vi "Similarities_to_colour_grid.vi"(11 "Array in":dbl[][](array[numeric])) -> (3 "Array out":u32[][](array[numeric]))   [LabVIEW 2016]
uses:
  <vilib>/Analysis/baseanly.llb/Mean (DBL).vi
  <vilib>/Analysis/NI_AALBase.lvlib
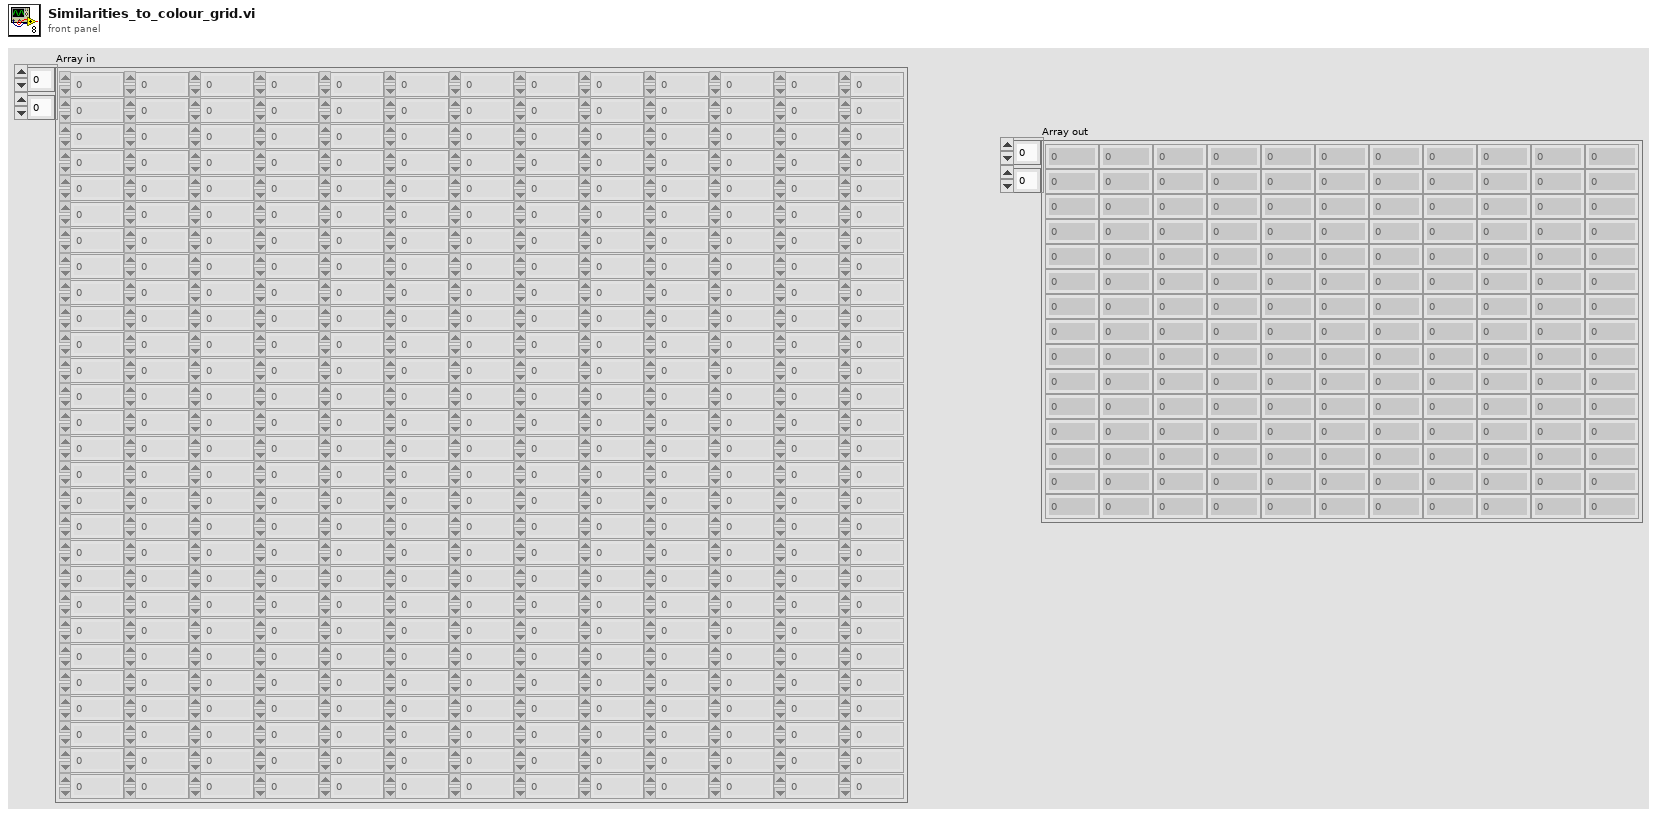
[diagram p1: front panel]
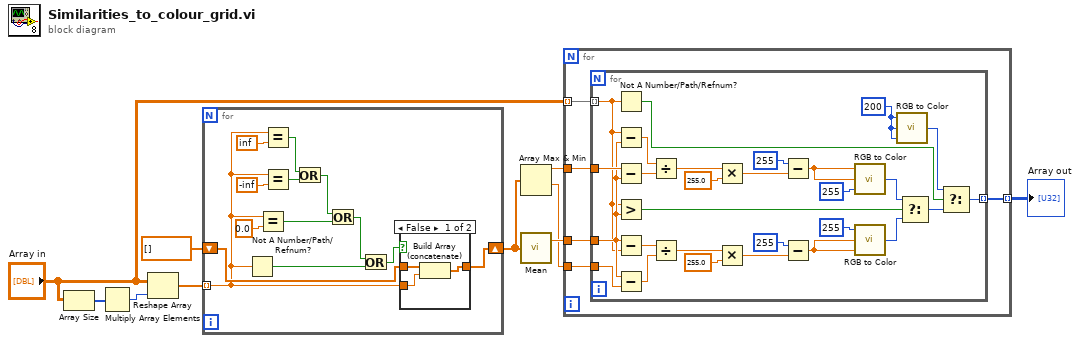
[diagram p0: block diagram]
diagram:
  n1 = Array Size(array="Array in") -> (size(s)=w2:i32[])
  n2 = Multiply Array Elements(1:w2) -> (0:w1:i32)
  n3 = Reshape Array("Array in", w1) -> (w6:dbl[])
  n4 = for {
    tunnel: w6 -> [w14] mode=indexing
    shift-right: [w21] -> w4
    shift-left: dbl[] [] ("output array") -> [w22]
    n5 = Not A Number/Path/Refnum?(number/path/refnum=w14) -> (NaN/Path/Refnum?=w13:bool)
    n6 = Equal?(x=w14, y=0.0) -> (x = y?=w16:bool)
    n7 = Equal?(x=w14, y=inf) -> (x = y?=w19:bool)
    n8 = Equal?(x=w14, y=-inf) -> (x = y?=w18:bool)
    n9 = Or(x=w19, y=w18) -> (x .or. y?=w17:bool)
    n10 = Or(x=w17, y=w16) -> (x .or. y?=w12:bool)
    n11 = Or(x=w12, y=w13) -> (x .or. y?=w11:bool)
    n12 = case shown="False" w11 {
      tunnel: w14 -> [w25 _]
      tunnel: w22 -> [w26 w27]
      tunnel: [w24 w27] -> w21
      frame False {
        n13 = Build Array (concatenate)(w26, w25) -> (w24:dbl[])
      }
      frame True {
      }
    }
  }
  n14 = Array Max & Min(array=w4) -> (max value=w9:dbl, min value=w8:dbl)  [unwired: 2 out]
  n15 = call-poly <vilib>:"Mean.vi"("X"=w4) -> ("mean"=w10:dbl)  [unwired: 1 out]
  n16 = for {
    tunnel: "Array in" -> [w32] mode=indexing
    tunnel: w10 -> [w31]
    tunnel: w9 -> [w30]
    tunnel: [w29] -> w7 mode=indexing
    tunnel: w8 -> [w28]
    n17 = for {
      tunnel: w32 -> [w38] mode=indexing
      tunnel: w31 -> [w52]
      tunnel: w30 -> [w58]
      tunnel: [w35] -> w29 mode=indexing
      tunnel: w28 -> [w51]
      w33 = u8 200 ("R")
      n18 = Not A Number/Path/Refnum?(number/path/refnum=w38) -> (NaN/Path/Refnum?=w36:bool)
      n19 = Subtract(x=w38, y=w52) -> (x-y=w59:dbl)
      n20 = Subtract(x=w58, y=w52) -> (x-y=w57:dbl)
      n21 = Greater?(x=w38, y=w52) -> (0:w60:bool)
      n22 = Subtract(x=w52, y=w38) -> (x-y=w53:dbl)
      n23 = Subtract(x=w52, y=w51) -> (x-y=w50:dbl)
      n24 = Divide(x=w59, y=w57) -> (x/y=w56:dbl)
      n25 = Divide(x=w53, y=w50) -> (x/y=w48:dbl)
      n26 = Multiply(x=w56, y=255.0) -> (x*y=w45:dbl)
      n27 = Multiply(x=w48, y=255.0) -> (x*y=w43:dbl)
      n28 = Subtract(x=u8 255 ("G"), y=w45) -> (x-y=w41:dbl)
      n29 = Subtract(x=u8 255 ("R"), y=w43) -> (x-y=w39:dbl)
      n30 = call <vilib>:"RGB to Color.vi"("B"=u8 255, "G"=w41, "R"=w41) -> ("Color"=w55:u32)
      n31 = call <vilib>:"RGB to Color.vi"("B"=w39, "G"=w39, "R"=u8 255 ("G")) -> ("Color"=w47:u32)
      n32 = call <vilib>:"RGB to Color.vi"("B"=w33, "G"=w33, "R"=w33) -> ("Color"=w34:u32)
      n33 = Select(t=w55, s=w60, f=w47) -> (s? t:f=w37:u32)
      n34 = Select(t=w34, s=w36, f=w37) -> (s? t:f=w35:u32)
    }
  }
  "Array out" <- w7
